vi "Difference.vi"(7 "error in (no error)":errorcluster, 8 "Compare to this JSON Object":string="{}", 10 "JSON Object":string="{}") -> (0 "error out":errorcluster, 3 "<JSON>":string caption="<JSON>Changes")   [LabVIEW 2021, in "jsontext.facade.lvlib"]
doc: "Compares (\"Diffs\") a JSON Object to another JSON Object.\n\nReturns a reduced-size Object that includes only changed elements."
uses:
  jsontext.facade.lvlib
  jsontext/JSONtext.lvlib
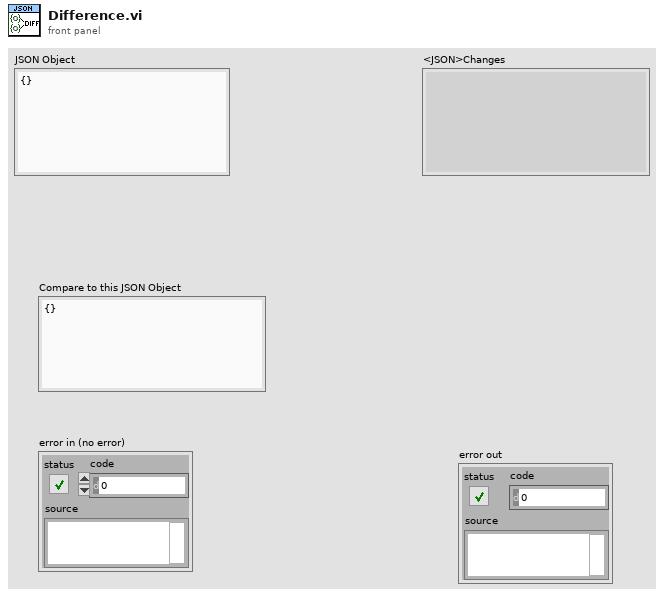
[diagram p1: front panel]
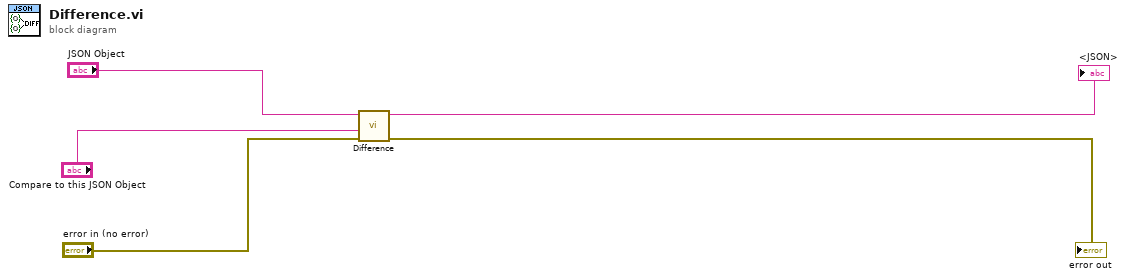
[diagram p0: block diagram]
diagram:
  n1 = call "Difference.vi"("error in (no error)"="error in (no error)", "Compare to this JSON Object"="Compare to this JSON Object", "JSON Object"="JSON Object") -> ("error out"=→"error out":errorcluster, "<JSON>"=→"<JSON>":string)  [unwired: 6 in]
